vi "VI Tree - picture.vi"() -> ()   [LabVIEW 2020]
panel:
  in  "Case Constant\n(See Context Help)":bool
  # "[OpenG VI Tags] ***Do Not Remove***"
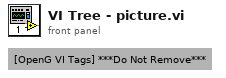
[diagram p1: front panel]
types:
  T1 = typedef "imagedata.ctl" = cluster{"image type":i32, "image depth":i32, "image":u8[], "mask":u8[], "colors":u32[], "Rectangle":cluster{"left":i16, "top":i16, "right":i16, "bottom":i16}}
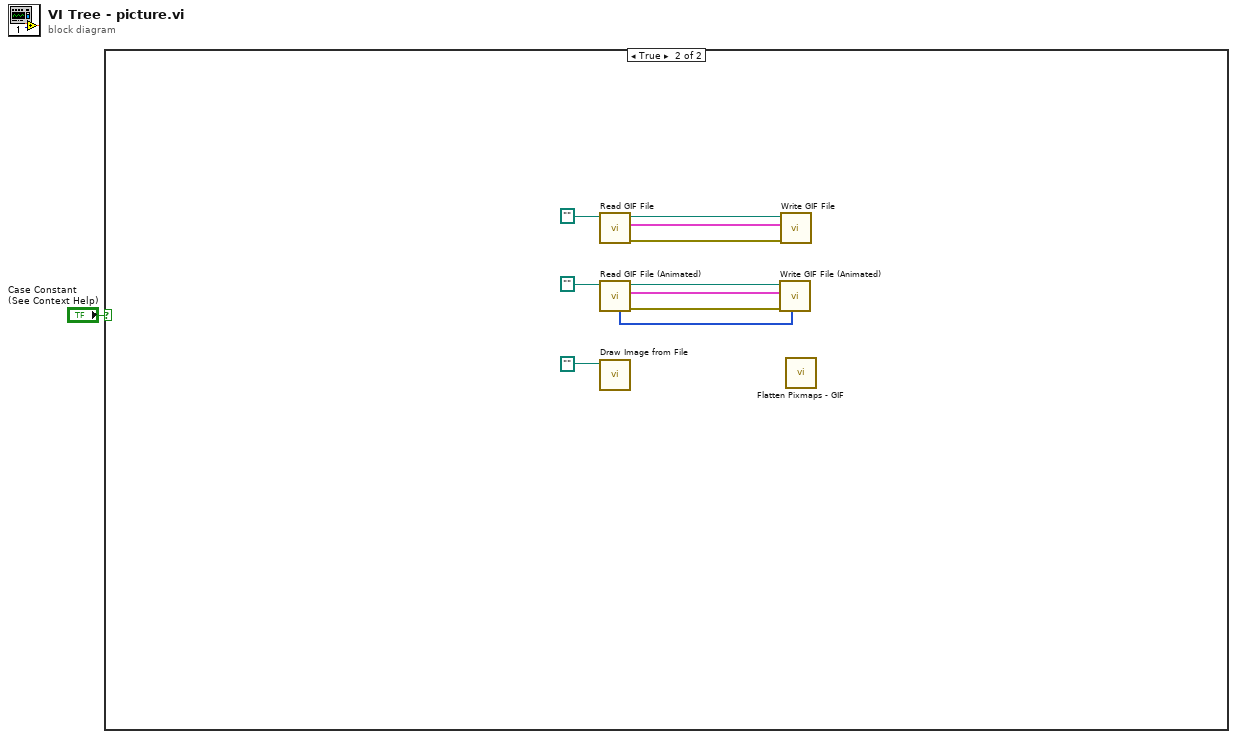
[diagram p0: block diagram]
diagram:
  n1 = case shown="True" "Case Constant\n(See Context Help)" {
    frame False {
    }
    frame True {
      n2 = call "Read GIF File.vi"("path to GIF file"=path "") -> ("error out"=w8:errorcluster, "image data"=w7:T1, "path"=w6:path)  [unwired: 8 in]
      n3 = call "Read GIF File (Animated).vi"("path to GIF file"=path "") -> ("error out"=w10:errorcluster, "images data"=w9:T1[], "path"=w5:path, "Delay (ms)"=w11:u32[])  [unwired: 6 in, 1 out]
      n4 = call "Draw Image from File.vi"("path to image file"=path "") -> ()  [unwired: 7 in, 4 out]
      n5 = call "Write GIF File (Animated).vi"("delay (ms)"=w11, "error in (no error)"=w10, "images data"=w9, "path to GIF file"=w5) -> ()  [unwired: 6 in, 2 out]
      n6 = call "Write GIF File.vi"("error in (no error)"=w8, "image data"=w7, "path to GIF file"=w6) -> ()  [unwired: 7 in, 2 out]
      n7 = call "Flatten Pixmaps - GIF.vi"() -> ()  [unwired: 11 in, 1 out]
    }
  }
